vi "getValue.vi"(8 "error in (no error)":errorcluster, 11 "tBSONDouble in":refnum<class "tBSONDouble.lvclass">) -> (0 "error out":errorcluster, 2 "Value":dbl, 3 "tBSONDouble out":refnum<class "tBSONDouble.lvclass">)   [LabVIEW 2013, in "BSON.lvlib" / "tBSONDouble.lvclass"]
uses:
  tBSONDouble.lvclass
  tBSONDouble.lvclass/tBSONDouble.ctl
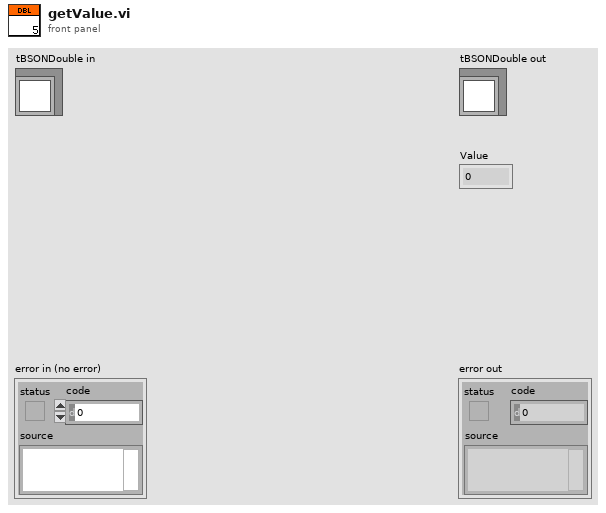
[diagram p1: front panel]
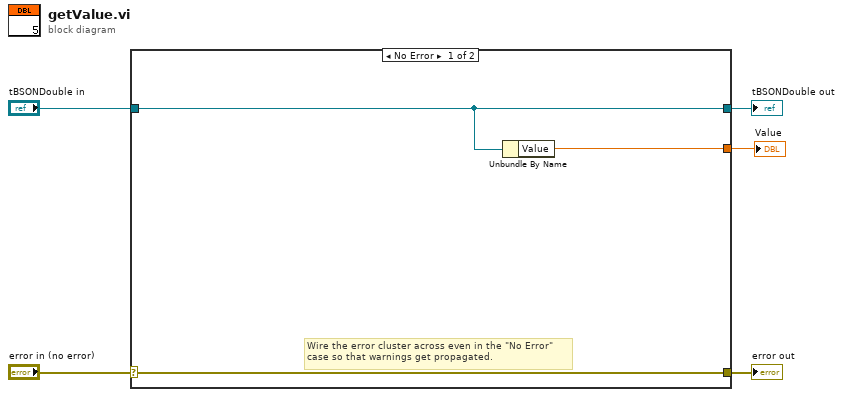
[diagram p0: block diagram]
diagram:
  n1 = case shown="No Error" "error in (no error)" {
    selector: "error in (no error)" -> [w8 w10]
    tunnel: [w8 w10] -> w4
    tunnel: [w7 w9] -> w2
    tunnel: "tBSONDouble in" -> [w7 w9]
    tunnel: [w6 _] -> w1
    frame No Error {
      # "Wire the error cluster across even in the \"No Error\"\ncase so that warnings get propagated."
      n2 = Unbundle By Name(w7) -> ("Value"=w6:dbl)
    }
    frame Error {
    }
  }
  "error out" <- w4
  "tBSONDouble out" <- w2
  "Value" <- w1
